vi "WinchMotor.vi"() -> ()   [LabVIEW 2013]
uses:
  State_Machine_Enum.ctl
  Robot Global Data.vi
panel:
  in  "WinchSpeed":dbl=0.2
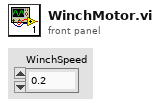
[diagram p1: front panel]
types:
  T1 = typedef "State_Machine_Enum.ctl" = enum16{"Idle", "Start", "Do", "Stop", "Init"}
  T2 = typedef "LoopDisable.ctl" = cluster{"Climb.vi":bool, "LauncherAngle.vi":bool, "Launcher.vi":bool, "ArmControl.vi":bool, "WinchMotor.vi":bool, "ReadDriveEncoder.vi":bool}
  T3 = typedef "WPI_MotorControlDeviceRef.ctl" = cluster{"DeviceStatus":errorcluster, "Type":enum16{"PWM", "CAN"}, "PWM":cluster{"Digital Module":T4, "PWM Channel":T5, "DeadBand":T6}, "CAN":cluster{"Device Number":u8, "Control Mode":T7, "Semaphore":T8, "Max Vout":dbl}, "Invert":bool, "TransformRef":T9, "InvTransformRef":T9}
  T4 = typedef "FPGA_TypedefDigitalModule.ctl" = enum16{"Digital Module 1", "Digital Module 2"}
  T5 = typedef "FPGA_DIOPWMChannel.ctl" = enum8{"PWM 1", "PWM 2", "PWM 3", "PWM 4", "PWM 5", "PWM 6", "PWM 7", "PWM 8", "PWM 9", "PWM 10", "Invalid"}
  T6 = typedef "WPI_PWMDeadband.ctl" = cluster{"Name":string, "maxPositivePwm":i32, "minPositivePwm":i32, "centerPwm":i32, "maxNegativePwm":i32, "minNegativePwm":i32, "angularRange":u16}
  T7 = typedef "WPI_CANJaguar_ControlMode.ctl" = enum8{"Percent VBus", "Current", "Speed", "Position", "Voltage"}
  T8 = typedef "Semaphore RefNum" = refnum<k1>
  T9 = typedef "WPI_PWMTransform_ConPane.ctl" = refnum<vi>
  T10 = typedef "WPI_DigitalInputDevRef.ctl" = cluster{"DevStatus":errorcluster, "DIO Channel":T11, "Digital Module":T4}
  T11 = typedef "FPGA_DIOChannel.ctl" = enum8{"DIO 1", "DIO 2", "DIO 3", "DIO 4", "DIO 5", "DIO 6", "DIO 7", "DIO 8", "DIO 9", "DIO 10", "DIO 11", "DIO 12", "DIO 13", "DIO 14", "Invalid"}
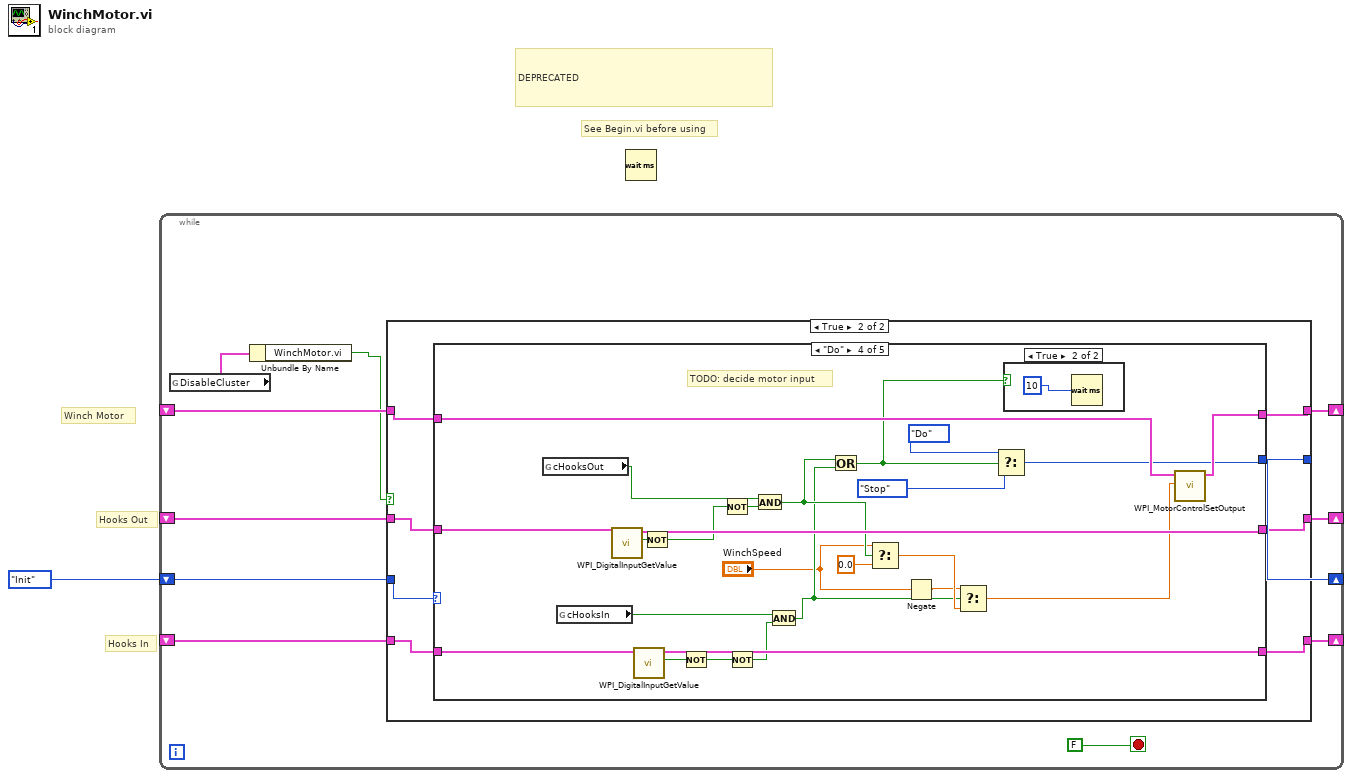
[diagram p0: block diagram]
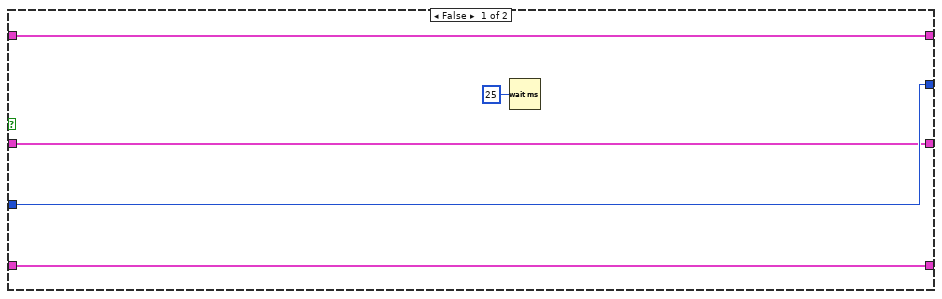
[diagram p2: hidden frame]
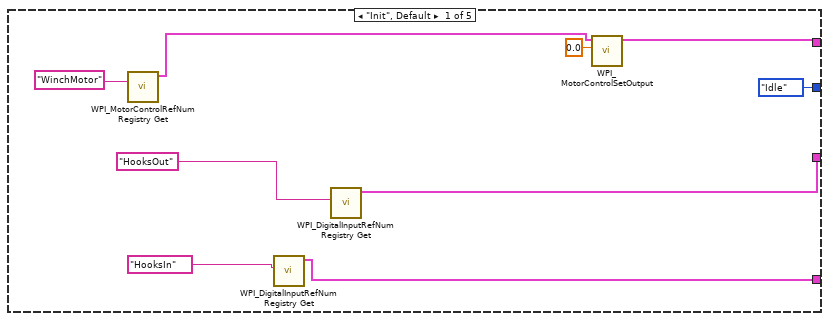
[diagram p3: hidden frame]
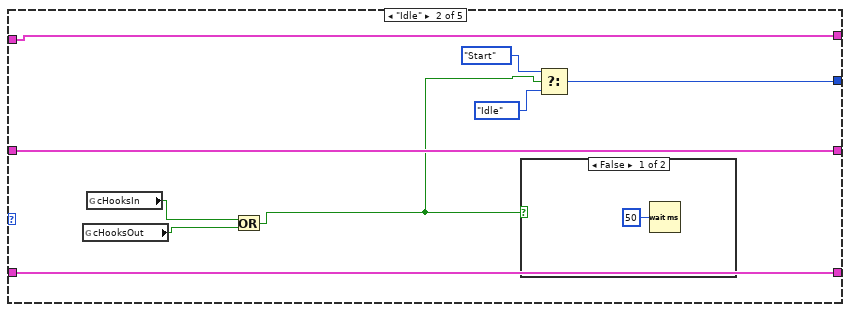
[diagram p4: hidden frame]
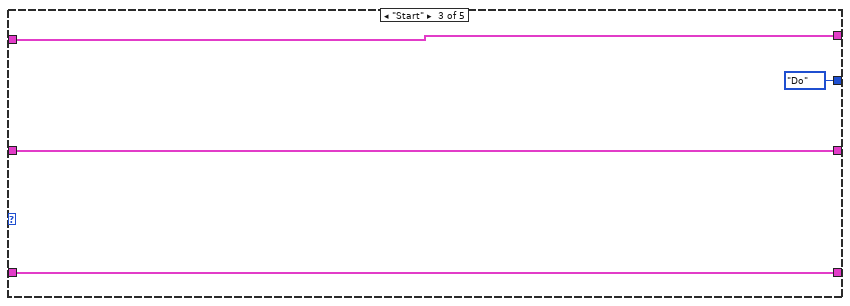
[diagram p6: hidden frame]
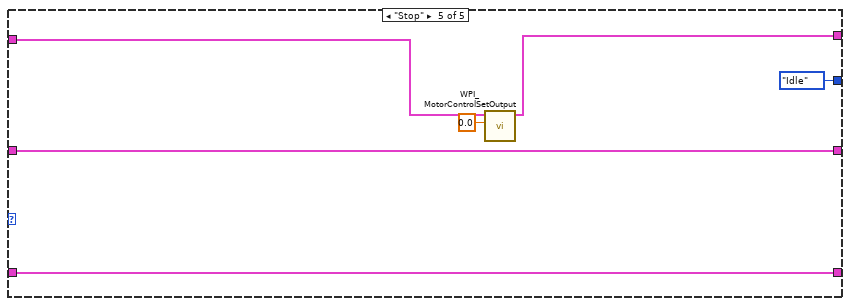
[diagram p8: hidden frame]
diagram:
  # "See Begin.vi before using"
  # "DEPRECATED"
  # "Hooks In"
  # "Hooks Out"
  # "Winch Motor"
  n1 = while {
    shift-right: [w10] -> _
    shift-left: _ -> [w11]
    shift-right: [w9] -> _
    shift-left: _ -> [w6]
    shift-right: [w8] -> _
    shift-left: _ -> [w7]
    shift-right: [w4] -> _
    shift-left: State_Machine_Enum."Init" ("State") -> [w5]
    stop <- FALSE stop-if-true
    n2 = global read "Robot Global Data.vi" "DisableCluster"() -> (w3:T2)
    n3 = Unbundle By Name(w3) -> ("WinchMotor.vi"=w2:bool)
    n4 = case shown="True" w2 {
      tunnel: w11 -> [w17 w25]
      tunnel: [w17 w24] -> w10
      tunnel: [w15 w23] -> w9
      tunnel: [w14 w22] -> w8
      tunnel: w7 -> [w14 w21]
      tunnel: w6 -> [w15 w20]
      tunnel: w5 -> [w16 w19]
      tunnel: [w16 w18] -> w4
      frame False {
        n5 = Wait (ms)(milliseconds to wait=u32 25) -> ()  [unwired: 1 out]
      }
      frame True {
        n6 = case shown="\"Do\"" w19 {
          tunnel: w25 -> [_ w35 w47 w73 w77]
          tunnel: [w27 w35 w47 w72 w76] -> w24
          tunnel: [w31 w42 w46 w71 w79] -> w23
          tunnel: [w30 w41 w45 w70 w78] -> w22
          tunnel: w21 -> [_ w41 w45 w69 w78]
          tunnel: w20 -> [_ w42 w46 w68 w79]
          tunnel: [State_Machine_Enum."Idle" ("State") w43 State_Machine_Enum."Do" ("f") w65 State_Machine_Enum."Idle" ("State")] -> w18
          frame "Init", Default {
            n7 = call <vilib>:"WPI_MotorControlRefNum Registry Get.vi"("refnum name"="WinchMotor") -> ("MotorControlDevRef"=w26:T3)  [unwired: 9 in, 1 out]
            n8 = call <vilib>:"WPI_DigitalInputRefNum Registry Get.vi"("refnum name"="HooksIn") -> ("DigitalInputDevRef"=w30:T10)  [unwired: 9 in, 1 out]
            n9 = call <vilib>:"WPI_DigitalInputRefNum Registry Get.vi"("refnum name"="HooksOut") -> ("DigitalInputDevRef"=w31:T10)  [unwired: 9 in, 1 out]
            n10 = call <vilib>:"WPI_MotorControlSetOutput.vi"("Output"=0.0, "MotorControlDevRef"=w26) -> ("MotorControlDevRef"=w27:T3)  [unwired: 7 in, 2 out]
          }
          frame "Idle" {
            n11 = global read "Robot Global Data.vi" "cHooksOut"() -> (w39:bool)
            n12 = global read "Robot Global Data.vi" "cHooksIn"() -> (w40:bool)
            n13 = Or(x=w40, y=w39) -> (x .or. y?=w38:bool)
            n14 = case shown="False" w38 {
              frame False {
                n15 = Wait (ms)(milliseconds to wait=u32 50) -> ()  [unwired: 1 out]
              }
              frame True {
              }
            }
            n16 = Select(t=State_Machine_Enum."Start" ("f"), s=w38, f=State_Machine_Enum."Idle") -> (s? t:f=w43:T1)
          }
          frame "Start" {
          }
          frame "Do" {
            # "TODO: decide motor input"
            n17 = global read "Robot Global Data.vi" "cHooksOut"() -> (w61:bool)
            n18 = global read "Robot Global Data.vi" "cHooksIn"() -> (w62:bool)
            n19 = call <vilib>:"WPI_DigitalInputGetValue.vi"("DigitalInputDevRef"=w68) -> ("Value"=w60:bool, "DigitalInputDevRef"=w71:T10)  [unwired: 8 in, 1 out]
            n20 = call <vilib>:"WPI_DigitalInputGetValue.vi"("DigitalInputDevRef"=w69) -> ("Value"=w64:bool, "DigitalInputDevRef"=w70:T10)  [unwired: 8 in, 1 out]
            n21 = Not(x=w60) -> (.not. x?=w50:bool)
            n22 = Not(x=w64) -> (.not. x?=w49:bool)
            n23 = Not(x=w50) -> (.not. x?=w59:bool)
            n24 = Not(x=w49) -> (.not. x?=w63:bool)
            n25 = And(x=w61, y=w59) -> (x .and. y?=w55:bool)
            n26 = And(x=w62, y=w63) -> (x .and. y?=w54:bool)
            n27 = Or(x=w55, y=w54) -> (x .or. y?=w53:bool)
            n28 = Select(t="WinchSpeed", s=w55, f=0.0) -> (s? t:f=w57:dbl)
            n29 = Negate(x="WinchSpeed") -> (-x=w52:dbl)
            n30 = Select(t=w52, s=w54, f=w57) -> (s? t:f=w56:dbl)
            n31 = Select(t=State_Machine_Enum."Do" ("State"), s=w53, f=State_Machine_Enum."Stop" ("State")) -> (s? t:f=w65:T1)
            n32 = case shown="True" w53 {
              frame False {
              }
              frame True {
                n33 = Wait (ms)(milliseconds to wait=u32 10) -> ()  [unwired: 1 out]
              }
            }
            n34 = call <vilib>:"WPI_MotorControlSetOutput.vi"("Output"=w56, "MotorControlDevRef"=w73) -> ("MotorControlDevRef"=w72:T3)  [unwired: 7 in, 2 out]
          }
          frame "Stop" {
            n35 = call <vilib>:"WPI_MotorControlSetOutput.vi"("Output"=0.0, "MotorControlDevRef"=w77) -> ("MotorControlDevRef"=w76:T3)  [unwired: 7 in, 2 out]
          }
        }
      }
    }
  }
  n36 = Wait (ms)() -> ()  [unwired: 1 in, 1 out]
